vi "3-3.vi"() -> ()   [LabVIEW 2018]
panel:
  out "量化误差":dbl[](array[numeric])
  out "编码数组":digitaldata
  out "还原信号数组":dbl[](array[numeric])
  in  "参考电压Vref（V）":dbl=2.56
  in  "信号数组":dbl[](array[numeric])
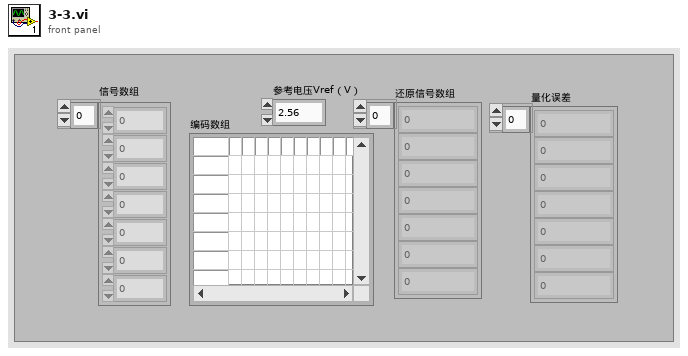
[diagram p1: front panel]
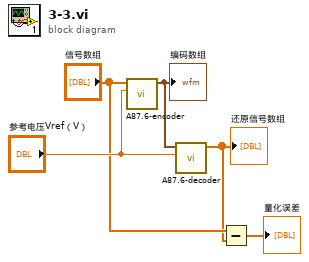
[diagram p0: block diagram]
diagram:
  n1 = call "A87.6-encoder.vi"("参考电压Vref（V）"="参考电压Vref（V）", "信号数组"="信号数组") -> ("编码数组"=w5:digitaldata)  [unwired: 9 in]
  "编码数组" <- w5
  n2 = call "A87.6-decoder.vi"("参考电压（V）"="参考电压Vref（V）", "编码数组"=w5) -> ("还原信号数组"=w2:dbl[])  [unwired: 9 in]
  "还原信号数组" <- w2
  n3 = Subtract(x="信号数组", y=w2) -> (x-y=→"量化误差":dbl[])
